vi "34970 Conf Scaling+.vi"(0 "VISA session":refnum<visa-resource-name>, 1 "Enable/Disable (T:Enable)":bool=TRUE, 2 "Set/Check (F:Set)":bool, 3 "m&b Fmt Str":string="%.;%0.6e", 5 "Gain (1)":dbl=1.0 min=-1000000000000.0 max=1000000000000.0 format="%.6f", 7 "Offset (0)":dbl min=-1000000000000.0 max=1000000000000.0 format="%.6f", 9 "Units(empty)":string, 11 "error in (no error)":errorcluster, 12 "Check (0:Gain)":enum16{"Gain", "Offset", "Status", "Units"}(ring), 13 "Channel List(empty)":string) -> (4 "dup VISA session":refnum<visa-resource-name>, 8 "Configuration?":string, 15 "error out":errorcluster)   [LabVIEW 2020]
doc: "This VI allows you to control or check measurement scaling and units. For example, you can add a gain and offset to certain channels' readings. You can also add a custom unit label."
panel:
  # "Check\nSet"
  # "Enable\nDisable"
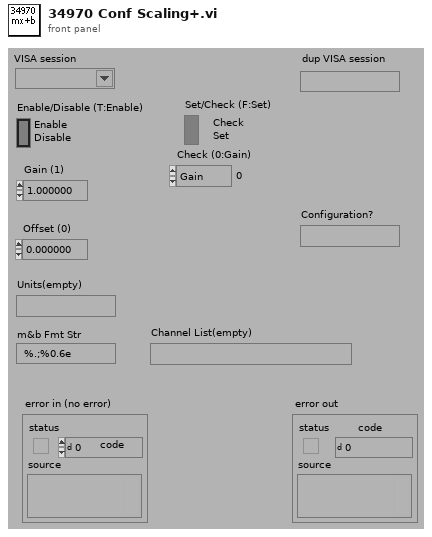
[diagram p1: front panel]
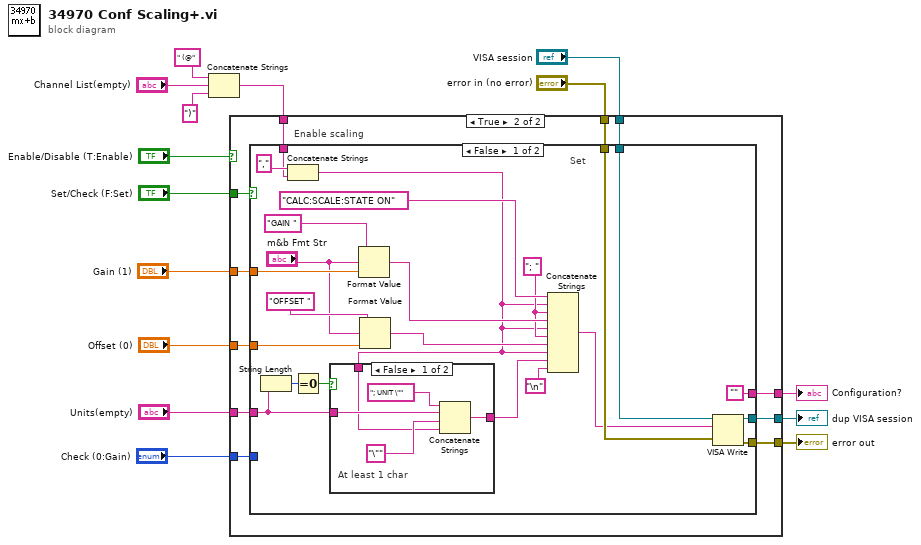
[diagram p0: block diagram]
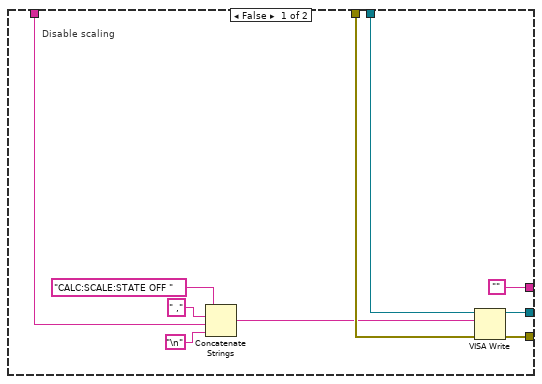
[diagram p2: hidden frame]
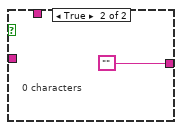
[diagram p3: hidden frame]
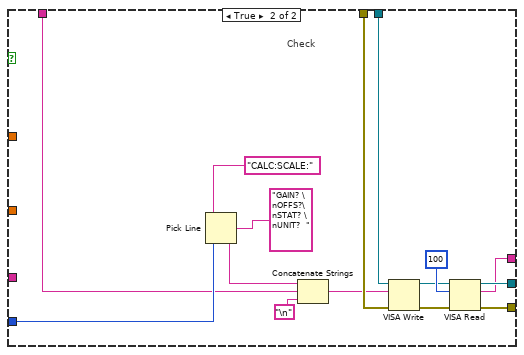
[diagram p4: hidden frame]
diagram:
  n1 = Concatenate Strings(" (@", "Channel List(empty)", ")") -> (w12:string)
  n2 = case shown="True" "Enable/Disable (T:Enable)" {
    tunnel: w12 -> [w19 w35]
    tunnel: "Check (0:Gain)" -> [_ w31]
    tunnel: "Set/Check (F:Set)" -> [_ w36]
    tunnel: "Gain (1)" -> [_ w34]
    tunnel: "Offset (0)" -> [_ w33]
    tunnel: "Units(empty)" -> [_ w32]
    tunnel: "error in (no error)" -> [w21 w30]
    tunnel: "VISA session" -> [w20 w29]
    tunnel: [w23 w28] -> w3
    tunnel: [w24 w27] -> w2
    tunnel: ["" w26] -> w1
    frame False {
      # "Disable scaling"
      n3 = Concatenate Strings("CALC:SCALE:STATE OFF ", " ,", w19, "\n") -> (w17:string)
      n4 = VISA Write(VISA resource name=w20, write buffer=w17, error in (no error)=w21) -> (VISA resource name out=w23:refnum<visa-resource-name>, error out=w24:errorcluster)  [unwired: 1 out]
    }
    frame True {
      # "Enable scaling"
      n5 = case shown="False" w36 {
        tunnel: w35 -> [w58 w77]
        tunnel: w34 -> [w57 _]
        tunnel: w33 -> [w54 _]
        tunnel: w32 -> [w43 _]
        tunnel: w31 -> [_ w78]
        tunnel: w30 -> [w50 w72]
        tunnel: w29 -> [w49 w71]
        tunnel: [w48 w70] -> w28
        tunnel: [w47 w69] -> w27
        tunnel: ["" w68] -> w26
        frame False {
          w42 = "; "
          # "Set"
          n6 = String Length(string=w43) -> (length=w45:i32)
          n7 = Concatenate Strings(",", w58) -> (w41:string)
          n8 = Equal To 0?(x=w45) -> (x = 0?=w44:bool)
          n9 = case shown="False" w44 {
            tunnel: w43 -> [w62 _]
            tunnel: [w63 ""] -> w40
            tunnel: w41 -> [w60 _]
            frame False {
              # "At least 1 char"
              n10 = Concatenate Strings("; UNIT \"", w62, "\"", w60) -> (w63:string)
            }
            frame True {
              # "0 characters"
            }
          }
          n11 = Format Value(string ("")="GAIN ", format string="m&b Fmt Str", value (0)=w57) -> (output string=w52:string)
          n12 = Format Value(string ("")="OFFSET ", format string="m&b Fmt Str", value (0)=w54) -> (output string=w51:string)
          n13 = Concatenate Strings("CALC:SCALE:STATE ON", w41, w42, w52, w41, w42, w51, w41, w40, "\n") -> (w38:string)
          n14 = VISA Write(VISA resource name=w49, write buffer=w38, error in (no error)=w50) -> (VISA resource name out=w48:refnum<visa-resource-name>, error out=w47:errorcluster)  [unwired: 1 out]
        }
        frame True {
          # "Check"
          n15 = Pick Line(string ("")="CALC:SCALE:", multi-line string="GAIN? \nOFFS?\nSTAT? \nUNIT?  ", line index=w78) -> (output string=w76:string)
          n16 = Concatenate Strings(w76, w77, "\n") -> (w66:string)
          n17 = VISA Write(VISA resource name=w71, write buffer=w66, error in (no error)=w72) -> (VISA resource name out=w74:refnum<visa-resource-name>, error out=w73:errorcluster)  [unwired: 1 out]
          n18 = VISA Read(VISA resource name=w74, byte count=u32 100 ("byte count (0)"), error in (no error)=w73) -> (VISA resource name out=w70:refnum<visa-resource-name>, read buffer=w68:string, error out=w69:errorcluster)  [unwired: 1 out]
        }
      }
    }
  }
  "dup VISA session" <- w3
  "error out" <- w2
  "Configuration?" <- w1
